vi "Assert Log Folder Is Empty.vi"(8 "error in":errorcluster, 9 "message on error":string="Log directory is not empty", 10 "directory":path=path "C:/logs/EDL2-archive/EDL Log2.tdms", 11 "Embedded Data Logger System Tests in":refnum<class "Embedded Data Logger Windows System Tests.lvclass">) -> (0 "error out":errorcluster, 3 "Embedded Data Logger System Tests out":refnum<class "Embedded Data Logger Windows System Tests.lvclass">)   [LabVIEW 2027, in "Embedded Data Logger Windows System Tests.lvclass"]
uses:
  Embedded Data Logger Windows System Tests.lvclass
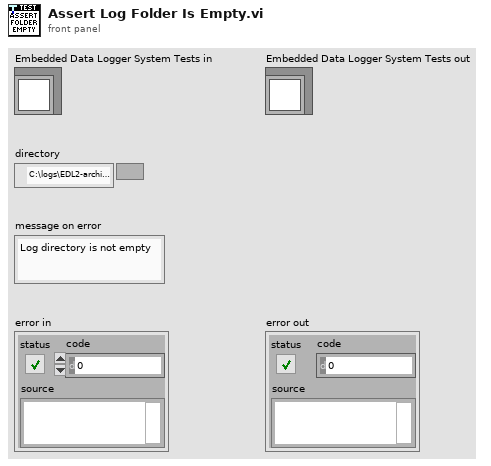
[diagram p1: front panel]
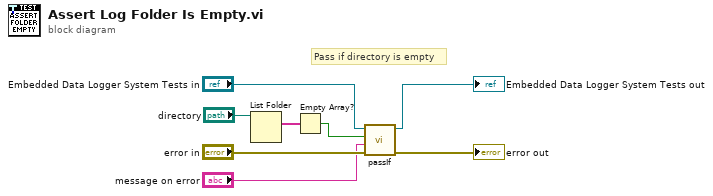
[diagram p0: block diagram]
diagram:
  # "Pass if directory is empty"
  n1 = List Folder(path="directory") -> (filenames=w3:string[])  [unwired: 3 in, 3 out]
  n2 = Empty Array?(array=w3) -> (empty?=w2:bool)
  n3 = call-dynamic "passIf.vi"("error in (no error)"="error in", "message (\"\")"="message on error", "pass"=w2, "TestCase in"="Embedded Data Logger System Tests in") -> ("error out"=→"error out":errorcluster, "TestCase out"=→"Embedded Data Logger System Tests out":refnum<class "Embedded Data Logger Windows System Tests.lvclass">)  [unwired: 6 in]
